vi "MinSec String.vi"(1 "Seconds":u32) -> (0 "MinSec string":string)   [LabVIEW 2020]
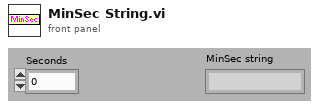
[diagram p1: front panel]
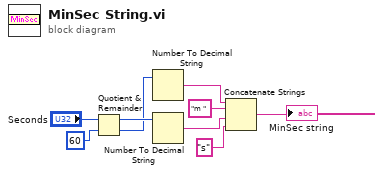
[diagram p0: block diagram]
diagram:
  n1 = Quotient & Remainder(x="Seconds", y=u32 60) -> (x-y*floor(x/y)=w7:u32, floor(x/y)=w6:u32)
  n2 = Number To Decimal String(number=w6) -> (decimal integer string=w5:string)  [unwired: 1 in]
  n3 = Number To Decimal String(number=w7) -> (decimal integer string=w4:string)  [unwired: 1 in]
  n4 = Concatenate Strings(w5, "m ", w4, "s") -> (→"MinSec string":string)
